vi "joint_final1.vi"(10 "Kinect 2":dbl[](array[numeric]), 11 "Kinect 1":dbl[](array[numeric])) -> (3 "Joint":dbl)   [LabVIEW 2016]
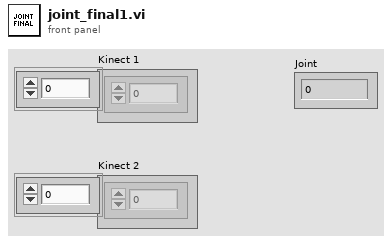
[diagram p1: front panel]
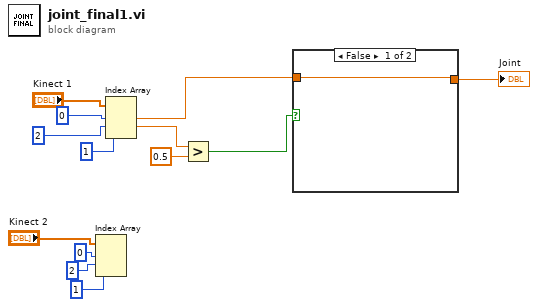
[diagram p0: block diagram]
diagram:
  n1 = Index Array(array="Kinect 2", index #1=0 ("index"), index #2=2 ("index"), index #3=1 ("index")) -> ()  [unwired: 3 out]
  n2 = Index Array(array="Kinect 1", index #1=0 ("index"), index #2=2 ("index"), index #3=1 ("index")) -> (element #1=w2:dbl, element #2=w1:dbl)  [unwired: 1 out]
  n3 = Greater?(x=w1, y=0.5) -> (0:w4:bool)
  n4 = case shown="False" w4 {
    tunnel: [w14 w15] -> w3
    tunnel: w2 -> [w14 w15]
    frame False {
    }
    frame True {
    }
  }
  "Joint" <- w3
